vi "Example - Authenticate using ticket.vi"() -> ()   [LabVIEW 2020, in "wamplv.lvlib"]
uses:
  wamplv.lvlib
  WAMP Client/WAMP Client.lvclass/WAMP Client.ctl
  WAMP Client/API/WAMP/Publish.vi/5e405bcd-0c6d-46be-a87b-06ec174a83c2.vi
  WAMP Client/API/WAMP/Publish (async).vi
  WAMP Client/Private/SubVIs/Raise Internal Message.vi
  WAMP Client/API/WAMP/Publish (async).vi/56cb05c7-ccfa-42e5-a428-2bd237dbc257.vi
  WAMP Client/Private/Authentication/Add Ticket authenticator.vi
  <vilib>/Utility/error.llb/Error Cluster From Error Code.vi
  WAMP Client/WAMP Client.lvclass
panel:
  in  "Ticket (e.g. password)":string="secret2"
  in  "Authorisation ID (e.g.username)":string="username"
  in  "Arguments":string
  in  "Topic URI":string="test.topic"
  in  "Realm":string="private_realm"
  in  "Router URL":string="ws://192.168.1.10:55555/"
  # "Example: authenticate with ticket and publish"
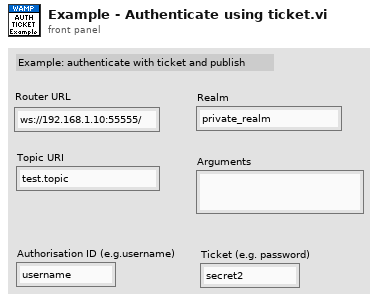
[diagram p1: front panel]
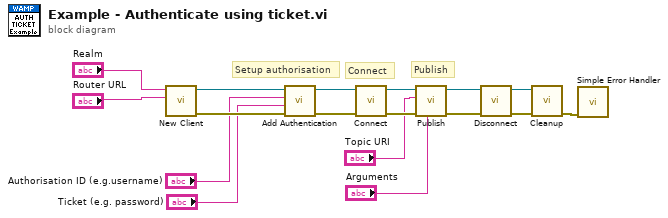
[diagram p0: block diagram]
diagram:
  # "Setup authorisation"
  # "Publish"
  # "Connect"
  n1 = call "New Client.vi"("Address"="Router URL", "Realm"="Realm") -> ("error out"=w5:errorcluster, "WAMP client out"=w6:refnum<class "WAMP Client.lvclass">)  [unwired: 8 in]
  n2 = call-poly "Add Authentication.vi"("error in (no error)"=w5, "Secret"="Ticket (e.g. password)", "Authentication ID"="Authorisation ID (e.g.username)", "WAMP Client in"=w6) -> ("error out"=w3:errorcluster, "WAMP Client out"=w4:refnum<class "WAMP Client.lvclass">)  [unwired: 6 in]
  n3 = call "Connect.vi"("error in"=w3, "WAMP Client in"=w4) -> ("error out"=w10:errorcluster, "WAMP Client out"=w12:refnum<class "WAMP Client.lvclass">)  [unwired: 8 in]
  n4 = call "Publish.vi"("Arguments"="Arguments", "Error in"=w10, "Topic"="Topic URI", "WAMP Client in"=w12) -> ("Error out"=w9:errorcluster, "WAMP Client out"=w11:refnum<class "WAMP Client.lvclass">)  [unwired: 5 in, 1 out]
  n5 = call-dynamic "Disconnect.vi"("error in"=w9, "WAMP Client in"=w11) -> ("error out"=w13:errorcluster, "WAMP Client out"=w15:refnum<class "WAMP Client.lvclass">)  [unwired: 8 in]
  n6 = call-dynamic "Cleanup.vi"("error in"=w13, "WAMP Client in"=w15) -> ("error out"=w14:errorcluster)  [unwired: 8 in, 1 out]
  n7 = call <vilib>:"Simple Error Handler.vi"("error in (no error)"=w14) -> ()  [unwired: 4 in, 5 out]
